vi "mean1 (SubVI).vi"(10 "mMean":i32=64, 11 "detected amplitude":dbl) -> (2 "size(s)":i32, 3 "mean":dbl)   [LabVIEW 2017]
uses:
  <vilib>/Analysis/baseanly.llb/Mean (DBL).vi
  <vilib>/Analysis/NI_AALBase.lvlib
panel:
  in  "mean_AMP1_PE2 in":dbl[](array[numeric])
  in  "I_AMP1_PE1":i32
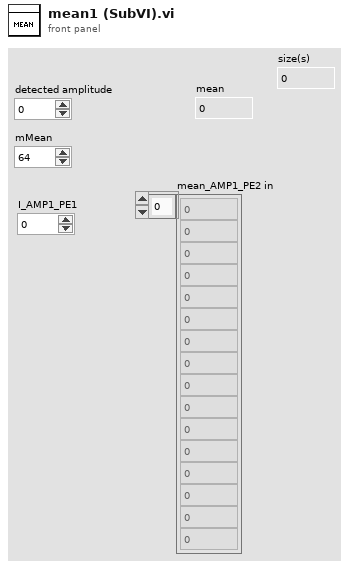
[diagram p1: front panel]
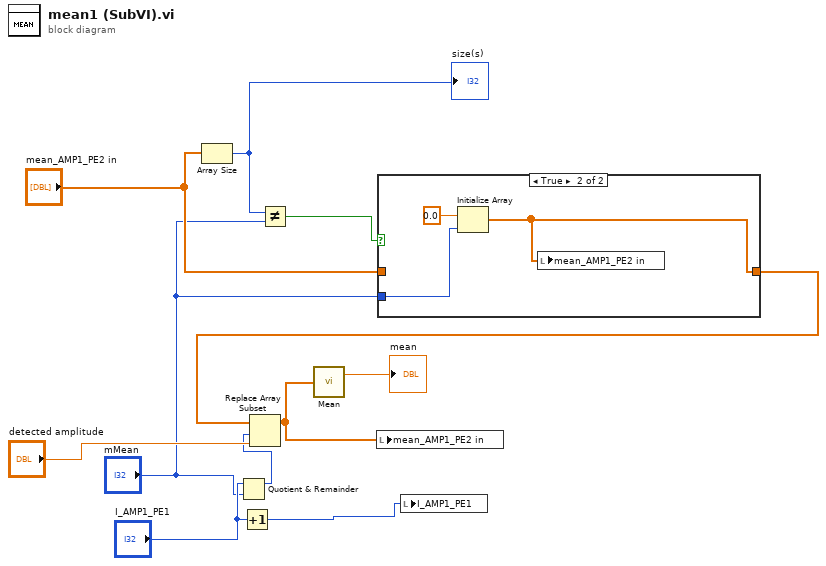
[diagram p0: block diagram]
diagram:
  n1 = Array Size(array="mean_AMP1_PE2 in") -> (size(s)=w5:i32)
  "size(s)" <- w5
  n2 = Quotient & Remainder(x="I_AMP1_PE1", y="mMean") -> (x-y*floor(x/y)=w8:i32)  [unwired: 1 out]
  n3 = Increment(x="I_AMP1_PE1") -> (x+1=w6:i32)
  n4 = Not Equal?(x=w5, y="mMean") -> (x != y?=w4:bool)
  n5 = case shown="True" w4 {
    tunnel: "mean_AMP1_PE2 in" -> [w12 _]
    tunnel: [w12 w13] -> w2
    tunnel: "mMean" -> [_ w14]
    frame False {
    }
    frame True {
      n6 = Initialize Array(0.0 ("element"), w14) -> (w13:dbl[])
      n7 = local write "mean_AMP1_PE2 in"(w13) -> ()
    }
  }
  n8 = Replace Array Subset(array=w2, new element="detected amplitude", index=w8) -> (w7:dbl[])
  n9 = call-poly <vilib>:"Mean.vi"("X"=w7) -> ("mean"=→"mean":dbl)  [unwired: 1 out]
  n10 = local write "mean_AMP1_PE2 in"(w7) -> ()
  n11 = local write "I_AMP1_PE1"(w6) -> ()
